vi "SHA-2-U32.vi"(7 "Type":T1, 8 "error in (no error)":errorcluster, 11 "Message":string="The quick brown fox jumps over the lazy dog") -> (0 "error out":errorcluster, 1 "ASCII formatted hash":string, 3 "binary string hash":string caption="binary string (hex formatted)")   [LabVIEW 2012, in "Encryption.lvlib"]
doc: "Performs a SHA-2 U32 hash action.\n\n(c) Ton Plomp, 2011\nTHIS SOFTWARE IS PROVIDED AS IS, AND ANY WARRANTY IS REJECTED"
uses:
  Encryption.lvlib
  SHA-2_U32_types.ctl
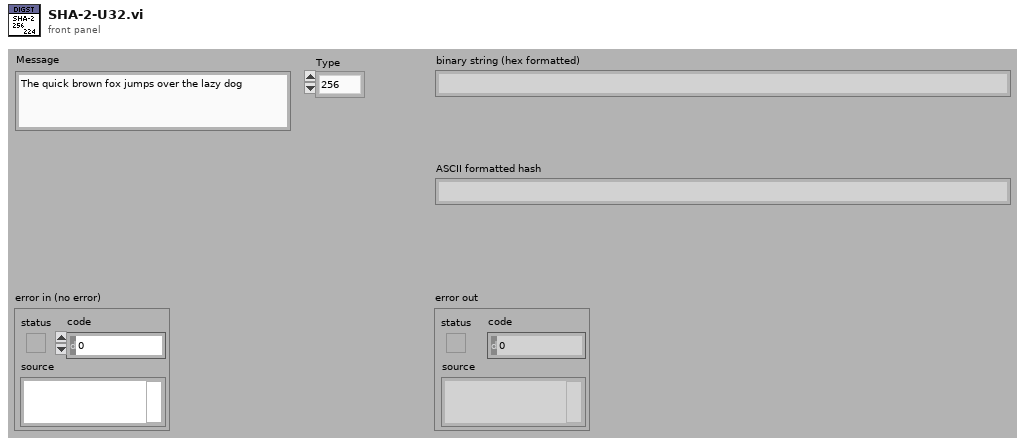
[diagram p1: front panel]
types:
  T1 = typedef "Encryption.lvlib/SHA-2_U32_types.ctl" = enum16{"256", "224"}
  T2 = enum16{"big-endian, network order", "native, host order", "little-endian"}
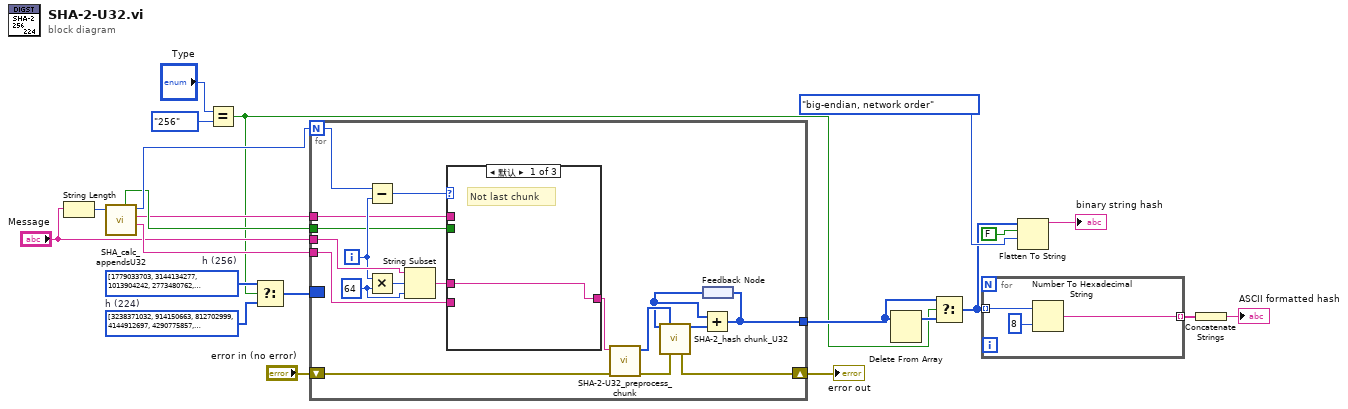
[diagram p0: block diagram]
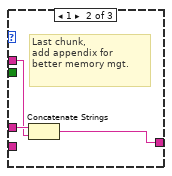
[diagram p2: hidden frame]
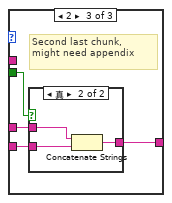
[diagram p3: hidden frame]
diagram:
  w5 = u32[] [3238371032, 914150663, 812702999, 4144912697, 4290775857, 1750603025, 1694076839, 3204075428]  # h (224)
  w7 = u32[] [1779033703, 3144134277, 1013904242, 2773480762, 1359893119, 2600822924, 528734635, 1541459225]  # h (256)
  n1 = String Length(string="Message") -> (length=w15:i32)
  n2 = call "SHA_calc_appendsU32.vi"("String length"=w15) -> ("Second last chunk"=w16:string, "Last Chunk"=w17:string, "Number of chunks"=w19:i32, "Double appends"=w18:bool)  [unwired: 7 in]
  n3 = Equal?(x="Type", y=SHA-2_U32_types."256" ("Type")) -> (x = y?=w1:bool)
  n4 = Select(t=w7, s=w1, f=w5) -> (s? t:f=w6:u32[])
  n5 = for {
    N: w19 -> [w37]
    tunnel: "Message" -> [w40]
    tunnel: w17 -> [w33]
    tunnel: [w24] -> w3
    border: w6 -> [_]
    tunnel: w18 -> [w30]
    tunnel: w16 -> [w29]
    shift-right: [w28] -> w13
    shift-left: "error in (no error)" -> [w27]
    i -> [w36]
    w38 = 64 ("x")
    n6 = Subtract(x=w37, y=w36) -> (x-y=w34:i32)
    n7 = Multiply(x=w36, y=w38) -> (x*y=w39:i32)
    n8 = String Subset(string=w40, offset (0)=w39, length (rest)=w38) -> (substring=w35:string)
    n9 = case shown="默认" w34 {
      tunnel: w35 -> [w41 w44 w48]
      tunnel: [w41 w42 w47] -> w31
      tunnel: w33 -> [_ w43 _]
      tunnel: w29 -> [_ _ w46]
      tunnel: w30 -> [_ _ w45]
      frame Default {
        # "Not last chunk"
      }
      frame 1 {
        # "Last chunk,\nadd appendix for\nbetter memory mgt."
        n10 = Concatenate Strings(w44, w43) -> (w42:string)
      }
      frame 2 {
        # "Second last chunk,\nmight need appendix"
        n11 = case shown="真" w45 {
          tunnel: w48 -> [w49 w52]
          tunnel: [w49 w51] -> w47
          tunnel: w46 -> [_ w50]
          frame False {
          }
          frame True {
            n12 = Concatenate Strings(w52, w50) -> (w51:string)
          }
        }
      }
    }
    n13 = call "SHA-2-U32_preprocess_chunk.vi"("error in (no error)"=w27, "Chunk in"=w31) -> ("error out"=w25:errorcluster, "Processed chunk out"=w26:u32[])  [unwired: 8 in]
    n14 = feedback #1() -> (w23:u32[])
    n15 = call "SHA-2_hash chunk_U32.vi"("h in"=w23, "Chunk"=w26, "error in (no error)"=w25) -> ("h out"=w32:u32[], "error out"=w28:errorcluster)  [unwired: 11 in]
    n16 = Add(x=w23, y=w32) -> (x+y=w24:u32[])
    n17 = feedback-in #1(w24) -> ()
  }
  "error out" <- w13
  n18 = Delete From Array(array=w3) -> (array with subset deleted=w2:u32[])  [unwired: 2 in, 1 out]
  n19 = Select(t=w3, s=w1, f=w2) -> (s? t:f=w4:u32[])
  n20 = for {
    tunnel: w4 -> [w55] mode=indexing
    tunnel: [w53] -> w11 mode=indexing
    n21 = Number To Hexadecimal String(1:i16 8 ("width (-)"), 2:w55) -> (0:w53:string)
  }
  n22 = Flatten To String(anything=w4, prepend array or string size? (T)=FALSE, byte order (0:big-endian, network order)=T2."big-endian, network order") -> (data string=→"binary string hash":string)  [unwired: 1 in, 2 out]
  n23 = Concatenate Strings(w11) -> (→"ASCII formatted hash":string)
